vi "encodeString.vi"(8 "error in (no error)":errorcluster, 10 "Variant":variant) -> (0 "error out":errorcluster, 2 "Array":u8[](array[numeric]) format="%.0x")   [LabVIEW 2016, in "MsgPack.lvlib"]
uses:
  MsgPack.lvlib
  <vilib>/Utility/Data Type/NI_Data Type.lvlib
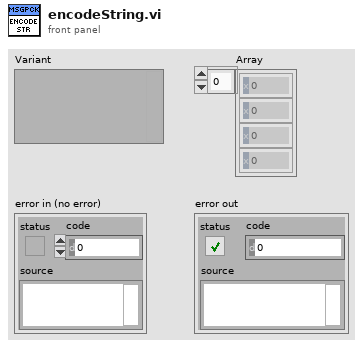
[diagram p1: front panel]
types:
  T1 = typedef "NI_Data Type.lvlib/Data Type.ctl" = enum8{"Invalid Type", "Void", "I8", "I16", "I32", "I64", "U8", "U16", "U32", "U64", "Single Float", "Double Float", "Extended Float", "Single Complex", "Double Complex", "Extended Complex", "Enum U8", "Enum U16", "Enum U32", "Enum U64", "Single Float With Unit", "Double Float With Unit", "Extended Float With Unit", "Single Complex with Unit", "Double Complex with Unit", "Extended Complex with Unit", "Boolean", "String", "Path", "Picture", "Tag", "Array", "Cluster", "Variant", "LV Variant", "Waveform", "Timestamp", "Digital Waveform", "Digital Data", "ExpressData", "Refnum", "External Data", "VI", "Poly VI", "LabVIEW Class Instance", "Fixed Point"}
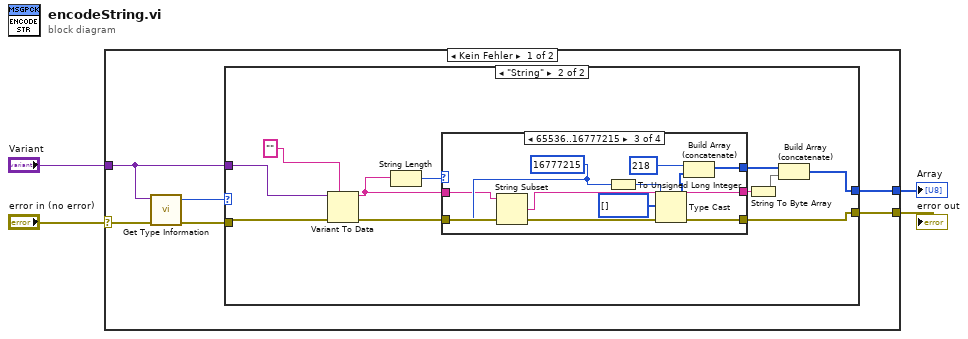
[diagram p0: block diagram]
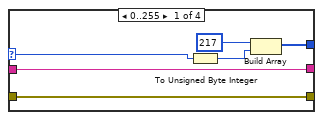
[diagram p3: hidden frame]
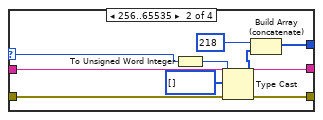
[diagram p4: hidden frame]
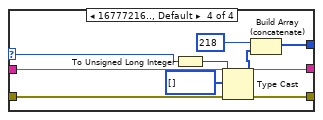
[diagram p5: hidden frame]
diagram:
  n1 = case shown="Kein Fehler" "error in (no error)" {
    selector: "error in (no error)" -> [w5 w54]
    tunnel: "Variant" -> [w8 _]
    tunnel: [w7 _] -> w3
    tunnel: [w6 w54] -> w2
    frame No Error {
      n2 = call <vilib>:"Get Type Information.vi"("error in (no error)"=w5, "Variant"=w8) -> ("error out"=w9:errorcluster, "Type"=w10:T1)  [unwired: 5 in, 3 out]
      n3 = case shown="\"String\"" w10 {
        tunnel: w9 -> [w11 w22]
        tunnel: w8 -> [_ w21]
        tunnel: [_ w13] -> w7
        tunnel: [w11 w12] -> w6
        frame "Invalid Type", Default {
        }
        frame "String" {
          n4 = Variant To Data(error in=w22, type="", Variant=w21) -> (data=w17:string, error out=w18:errorcluster)
          n5 = String Length(string=w17) -> (length=w19:i32)
          n6 = case shown="65536..16777215" w19 {
            selector: w19 -> [w24 w32 _ w49]
            tunnel: w18 -> [w28 w36 w45 w53]
            tunnel: [w28 w36 w45 w53] -> w12
            tunnel: [w26 w34 w37 w51] -> w14
            tunnel: w17 -> [w26 w34 w38 w51]
            tunnel: [w25 w33 w43 w50] -> w16
            frame 0..255 {
              n7 = To Unsigned Byte Integer(number=w24) -> (unsigned 8bit integer=w23:u8)
              n8 = Build Array(u8 217, w23) -> (w25:u8[])
            }
            frame 256..65535 {
              n9 = To Unsigned Word Integer(number=w32) -> (unsigned 16bit integer=w31:u16)
              n10 = Type Cast(type=u8[] [] ("appended array"), x=w31) -> (*(type *) &x=w29:u8[])
              n11 = Build Array (concatenate)(u8 218, w29) -> (w33:u8[])
            }
            frame 65536..16777215 {
              w39 = u32 16777215 ("number")
              n12 = String Subset(string=w38, length (rest)=w39) -> (substring=w37:string)  [unwired: 1 in]
              n13 = To Unsigned Long Integer(number=w39) -> (unsigned 32bit integer=w42:u32)
              n14 = Type Cast(type=u8[] [] ("appended array"), x=w42) -> (*(type *) &x=w40:u8[])
              n15 = Build Array (concatenate)(u8 218, w40) -> (w43:u8[])
            }
            frame 16777216.., Default {
              n16 = To Unsigned Long Integer(number=w49) -> (unsigned 32bit integer=w48:u32)
              n17 = Type Cast(type=u8[] [] ("appended array"), x=w48) -> (*(type *) &x=w46:u8[])
              n18 = Build Array (concatenate)(u8 218, w46) -> (w50:u8[])
            }
          }
          n19 = String To Byte Array(string=w14) -> (unsigned byte array=w15:u8[])
          n20 = Build Array (concatenate)(w16, w15) -> (w13:u8[])
        }
      }
    }
    frame Error {
    }
  }
  "Array" <- w3
  "error out" <- w2
